vi "Stopped.vi"(6 "Teller":refnum<class "Teller.lvclass">, 8 "Error in":errorcluster, 9 "Error":errorcluster, 10 "Actor":refnum<class "Actor.lvclass">, 11 "Base Actor in":refnum<class "Base Actor.lvclass">) -> (0 "Error out":errorcluster, 3 "Base Actor out":refnum<class "Base Actor.lvclass">)   [LabVIEW 2025, in "jettl.lvlib" / "Base jettl Actor.lvlib" / "Base Actor.lvlib" / "Base Actor.lvclass"]
uses:
  Base Actor.lvclass
  Base Actor.lvclass/Base Actor.ctl
  Stop jettl Msg/Stop/Stop.lvlib
  Actor/Actor.lvclass
  Attributes/Attributes.lvclass
  Teller/Teller.lvclass
  Stop jettl Msg/Stop/Call.vi
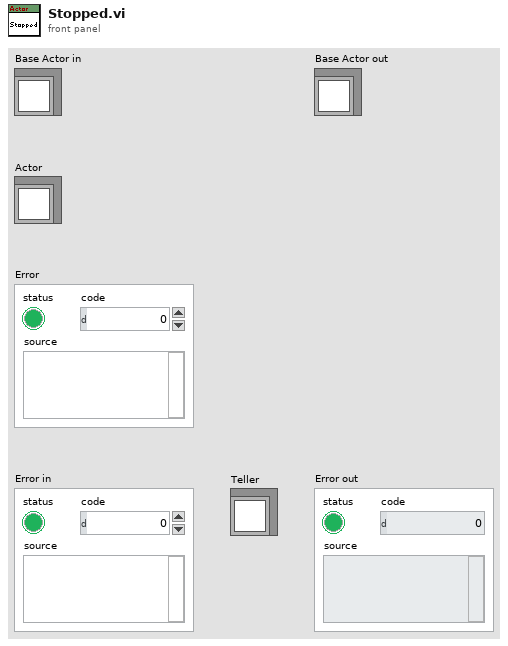
[diagram p1: front panel]
types:
  T1 = typedef "jettl.lvlib/Relation.ctl" = enum16{"Self", "Parent", "Child", "No Relation"}
  T2 = typedef "jettl.lvlib/All Child Attributes.ctl" = map{string, refnum<class "Attributes.lvclass">}
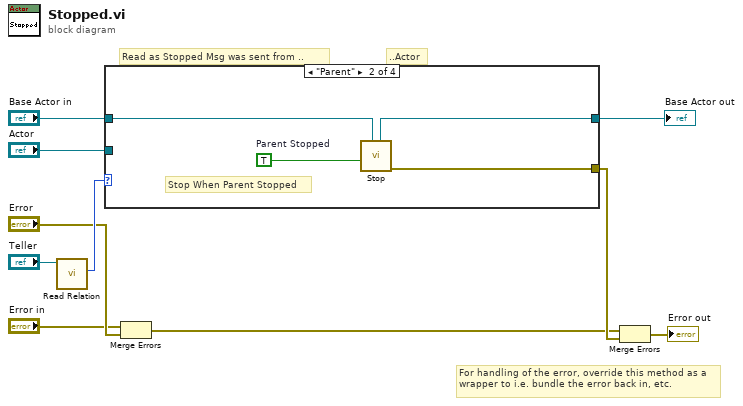
[diagram p0: block diagram]
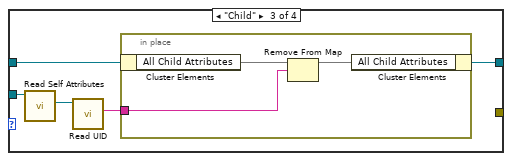
[diagram p3: hidden frame]
diagram:
  # "For handling of the error, override this method as a wrapper to i.e. bundle the error back in, etc."
  # "..Actor"
  # "Read as Stopped Msg was sent from .."
  n1 = call-dynamic "Read Relation.vi"("Teller in"="Teller") -> ("Relation"=w6:T1)  [unwired: 10 in]
  n2 = case shown="\"Parent\"" w6 {
    tunnel: "Base Actor in" -> [w11 w13 w19 w24]
    tunnel: [w11 w15 w16 w24] -> w10
    tunnel: "Actor" -> [_ _ w20 _]
    tunnel: [_ w14 _ _] -> w4
    frame "Self" {
      # "Case will not fundamentally execute"
    }
    frame "Parent" {
      w12 = TRUE  # Parent Stopped
      # "Stop When Parent Stopped"
      n3 = call-poly "Stop.vi"("Actor in"=w13, "Parent Stopped"=w12) -> ("Error out"=w14:errorcluster, "Actor out"=w15:refnum<class "Base Actor.lvclass">)  [unwired: 8 in]
    }
    frame "Child" {
      n4 = call-dynamic "Read Self Attributes.vi"("Actor in"=w20) -> ("Self Attributes"=w18:refnum<class "Attributes.lvclass">)  [unwired: 10 in]
      n5 = call-dynamic "Read UID.vi"("Attributes in"=w18) -> ("UID"=w17:string)  [unwired: 10 in]
      n6 = in-place {
        in-place-border: w17 -> [w21]
        n7 = in-place-cluster #1(w19) -> ("All Child Attributes"=w23:T2)
        n8 = Remove From Map(10:w21, 11:w23) -> (3:w22:T2)  [unwired: 2 out]
        n9 = in-place-cluster #1("All Child Attributes"=w22) -> (w16:refnum<class "Base Actor.lvclass">)
      }
    }
    frame "No Relation" {
      # "Case will not fundamentally execute"
    }
  }
  "Base Actor out" <- w10
  n10 = Merge Errors("Error in", "Error") -> (w2:errorcluster)
  n11 = Merge Errors(w2, w4) -> (→"Error out":errorcluster)
